vi "Visa read.vi"(8 "error in (no error)":errorcluster, 11 "VISA Refnum in":refnum<visa-resource-name>) -> (0 "error out":errorcluster, 2 "String":string, 3 "VISA Refnum out":refnum<visa-resource-name>)   [LabVIEW 2020, in "Cypress.lvclass"]
uses:
  Cypress.lvclass
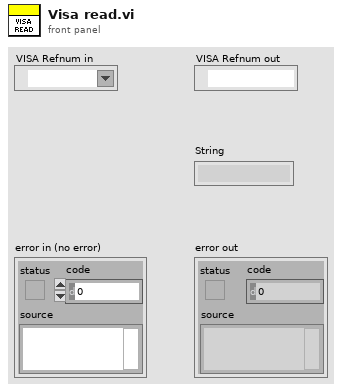
[diagram p1: front panel]
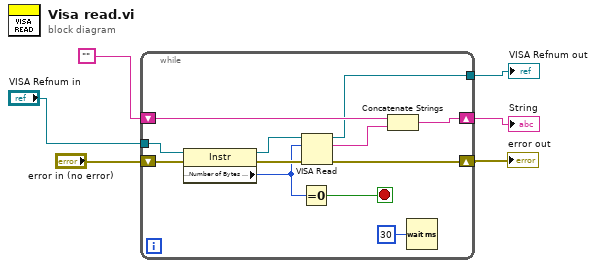
[diagram p0: block diagram]
diagram:
  n1 = while {
    shift-right: [w18] -> w3
    shift-left: "error in (no error)" -> [w17]
    shift-right: [w12] -> w4
    shift-left: "" -> [w13]
    tunnel: [w8] -> w5
    tunnel: "VISA Refnum in" -> [w7]
    stop <- w9 stop-if-true
    n2 = property class="Instr"(reference=w7, error in=w17) -> (reference out=w15:refnum<visa-resource-name>, error out=w16:errorcluster, "Serial Settings:Number of Bytes at Serial Port"=w10:u32)
    n3 = Equal To 0?(x=w10) -> (x = 0?=w9:bool)
    n4 = VISA Read(VISA resource name=w15, byte count=w10, error in (no error)=w16) -> (VISA resource name out=w8:refnum<visa-resource-name>, read buffer=w14:string, error out=w18:errorcluster)  [unwired: 1 out]
    n5 = Concatenate Strings(w13, w14) -> (w12:string)
    n6 = Wait (ms)(milliseconds to wait=u32 30) -> ()  [unwired: 1 out]
  }
  "error out" <- w3
  "String" <- w4
  "VISA Refnum out" <- w5
